vi "filter.hostToFpga.testRunner.vi"(6 "Request.Debug?":bool, 8 "error in":errorcluster, 9 "Watch.List":string[](array[string])=["AAPL"], 10 "Expected OrderBook.Command[]":T2[](array[typedef])=[{"type"=enum."AddOrder", "side"=66, "orderId "=3544385890602799695, "quantity"=20000, "symbol"=4702127773838213120, "price"=9050, "executed.qty"=0, "canceled.qty"=0, "remaining.qty"=0, "seconds"=0, "nanoseconds"=0, "Add"=FALSE, "Edit"=FALSE, "Remove"=FALSE, "seq no"=0, "recv.time"=0, "parse.time"=0}, {"type"=enum."AddOrder", "side"=66, "orderId "=3616443484640727631, "quantity"=20000, "symbol"=4702127773838213120, "price"=9050, "executed.qty"=0, "canceled.qty"=0, "remaining.qty"=0, "seconds"=0, "nanoseconds"=0, "Add"=FALSE, "Edit"=FALSE, "Remove"=FALSE, "seq no"=0, "recv.time"=0, "parse.time"=0}, {"type"=enum."AddOrder", "side"=66, "orderId "=3688501078678655567, "quantity"=20000, "symbol"=4702127773838213120, "price"=9050, "executed.qty"=0, "canceled.qty"=0, "remaining.qty"=0, "seconds"=0, "nanoseconds"=0, "Add"=FALSE, "Edit"=FALSE, "Remove"=FALSE, "seq no"=0, "recv.time"=0, "parse.time"=0}, {"type"=enum."AddOrder", "side"=66, "orderId "=3760558672716583503, "quantity"=20000, "symbol"=4702127773838213120, "price"=9050, "executed.qty"=0, "canceled.qty"=0, "remaining.qty"=0, "seconds"=0, "nanoseconds"=0, "Add"=FALSE, "Edit"=FALSE, "Remove"=FALSE, "seq no"=0, "recv.time"=0, "parse.time"=0}, {"type"=enum."AddOrder", "side"=66, "orderId "=3832616266754511439, "quantity"=20000, "symbol"=4702127773838213120, "price"=9050, "executed.qty"=0, "canceled.qty"=0, "remaining.qty"=0, "seconds"=0, "nanoseconds"=0, "Add"=FALSE, "Edit"=FALSE, "Remove"=FALSE, "seq no"=0, "recv.time"=0, "parse.time"=0}, {"type"=enum."AddOrder", "side"=66, "orderId "=3904673860792439375, "quantity"=20000, "symbol"=4702127773838213120, "price"=9050, "executed.qty"=0, "canceled.qty"=0, "remaining.qty"=0, "seconds"=0, "nanoseconds"=0, "Add"=FALSE, "Edit"=FALSE, "Remove"=FALSE, "seq no"=0, "recv.time"=0, "parse.time"=0}, {"type"=enum."AddOrder", "side"=66, "orderId "=3976731454830367311, "quantity"=20000, "symbol"=4702127773838213120, "price"=9050, "executed.qty"=0, "canceled.qty"=0, "remaining.qty"=0, "seconds"=0, "nanoseconds"=0, "Add"=FALSE, "Edit"=FALSE, "Remove"=FALSE, "seq no"=0, "recv.time"=0, "parse.time"=0}, {"type"=enum."AddOrder", "side"=66, "orderId "=4048789048868295247, "quantity"=20000, "symbol"=4702127773838213120, "price"=9050, "executed.qty"=0, "canceled.qty"=0, "remaining.qty"=0, "seconds"=0, "nanoseconds"=0, "Add"=FALSE, "Edit"=FALSE, "Remove"=FALSE, "seq no"=0, "recv.time"=0, "parse.time"=0}, {"type"=enum."AddOrder", "side"=66, "orderId "=4120846642906223183, "quantity"=20000, "symbol"=4702127773838213120, "price"=9050, "executed.qty"=0, "canceled.qty"=0, "remaining.qty"=0, "seconds"=0, "nanoseconds"=0, "Add"=FALSE, "Edit"=FALSE, "Remove"=FALSE, "seq no"=0, "recv.time"=0, "parse.time"=0}, {"type"=enum."AddOrder", "side"=66, "orderId "=4697307395209646671, "quantity"=20000, "symbol"=4702127773838213120, "price"=9050, "executed.qty"=0, "canceled.qty"=0, "remaining.qty"=0, "seconds"=0, "nanoseconds"=0, "Add"=FALSE, "Edit"=FALSE, "Remove"=FALSE, "seq no"=0, "recv.time"=0, "parse.time"=0}, {"type"=enum."AddOrder", "side"=66, "orderId "=4769364989247574607, "quantity"=20000, "symbol"=4702127773838213120, "price"=9050, "executed.qty"=0, "canceled.qty"=0, "remaining.qty"=0, "seconds"=0, "nanoseconds"=0, "Add"=FALSE, "Edit"=FALSE, "Remove"=FALSE, "seq no"=0, "recv.time"=0, "parse.time"=0}] {"symbol" format="%.0x"; "orderId" format="%.0x"; "side" format="%.0x"}, 11 "OrderBook.Commands.in":T2[](array[typedef]) {"symbol" format="%.0x"; "orderId" format="%.0x"; "side" format="%.0x"}) -> (0 "error out":errorcluster={"status"=TRUE, "code"=-61165, "source"="Open FPGA VI Reference in host.bats.parser.tester.vi"}, 1 "Data.Results.out":T4, 2 "Metadata.Results.out":T1)   [LabVIEW 2020]
uses:
  <vilib>/rvi/interface/nirviOpenFPGA/nirviOpenFPGA.xnode
  <vilib>/rvi/interface/nirviMethod/nirviMethod.xnode
  <vilib>/rvi/interface/nirviCloseFPGA/nirviCloseFPGA.xnode
  <vilib>/rvi/errors/niLvFpgaMergeErrorWithErrorCode.vi
  <vilib>/FPGAPlugInAG/Dynamic/niLvFpga_ReadFifo_Dynamic.vi
  <vilib>/rvi/interface/nirviReadWriteControl/nirviReadWriteControl.xnode
  <vilib>/rvi/interface/Simulation/niFpgaSimulationCallBeginRW.vi
  <vilib>/rvi/errors/niLvFpgaAdjustHostInterfaceError.vi
  NiFpgaLv.dll
  <vilib>/Utility/error.llb/Error Cluster From Error Code.vi
  <vilib>/FPGAPlugInAG/Dynamic/niLvFpga_WriteFifo_Dynamic.vi
  Market.Data.Common/host/fpganow.common.host.lvlib
  Market.Data.Common/fpga/orderbook.command.type.ctl
  Market.Data.Common/fpga/fpganow.common.fpga.lvlib
  Market.Data.Common/fpga/orderbook.command.ctl
  fpga/filter.test.vi
  <vilib>/FPGAPlugInAG/Dynamic/niLvFpga_Close_Dynamic.vi
  <vilib>/rvi/interface/RandomDataEmulation/nirviRandomDataOpen.vi
  <vilib>/rvi/interface/common/niFpgaCacheSessionInfoDynamic.vi
panel:
  in  "Metadata.Results":T1
  in  "Data.Results":T4
  out "Memory":u64[](array[numeric]) format="%.0x"
  out "HT-Filter.Commands.In":u64[](array[numeric])=[1, 66, 48, 20000, 4702127773838221344, 9050, 0, 0, 0, 0, 0, 0, 0, 0, 0, 0, 2, 66, 48, 0, 0, 9050, 200, 0, 0, 0, 0, 0, 0, 0, 0, 0, 5, 66, 48, 1400, 6076284164848492576, 9050, 0, 0, 0, 0, 0, 0, 0, 0, 0, 0] format="%.0x"
  out "GetState":u64[](array[numeric]) format="%.0x"
  out "Match.Details":bool[][](array[boolean])
  out "Debug.Normal.out":u64[](array[numeric]) format="%.0x"
  out "Failures.Count":i32
  out "Passed":bool
  out "OrderBook.Commands.out":T2[](array[typedef]) {"symbol" format="%.0x"; "orderId" format="%.0x"; "side" format="%.0x"}
  out "Data.size":i32
  in  "Execute?":bool=TRUE
  out "Data.out":u64[](array[numeric]) format="%.0x"
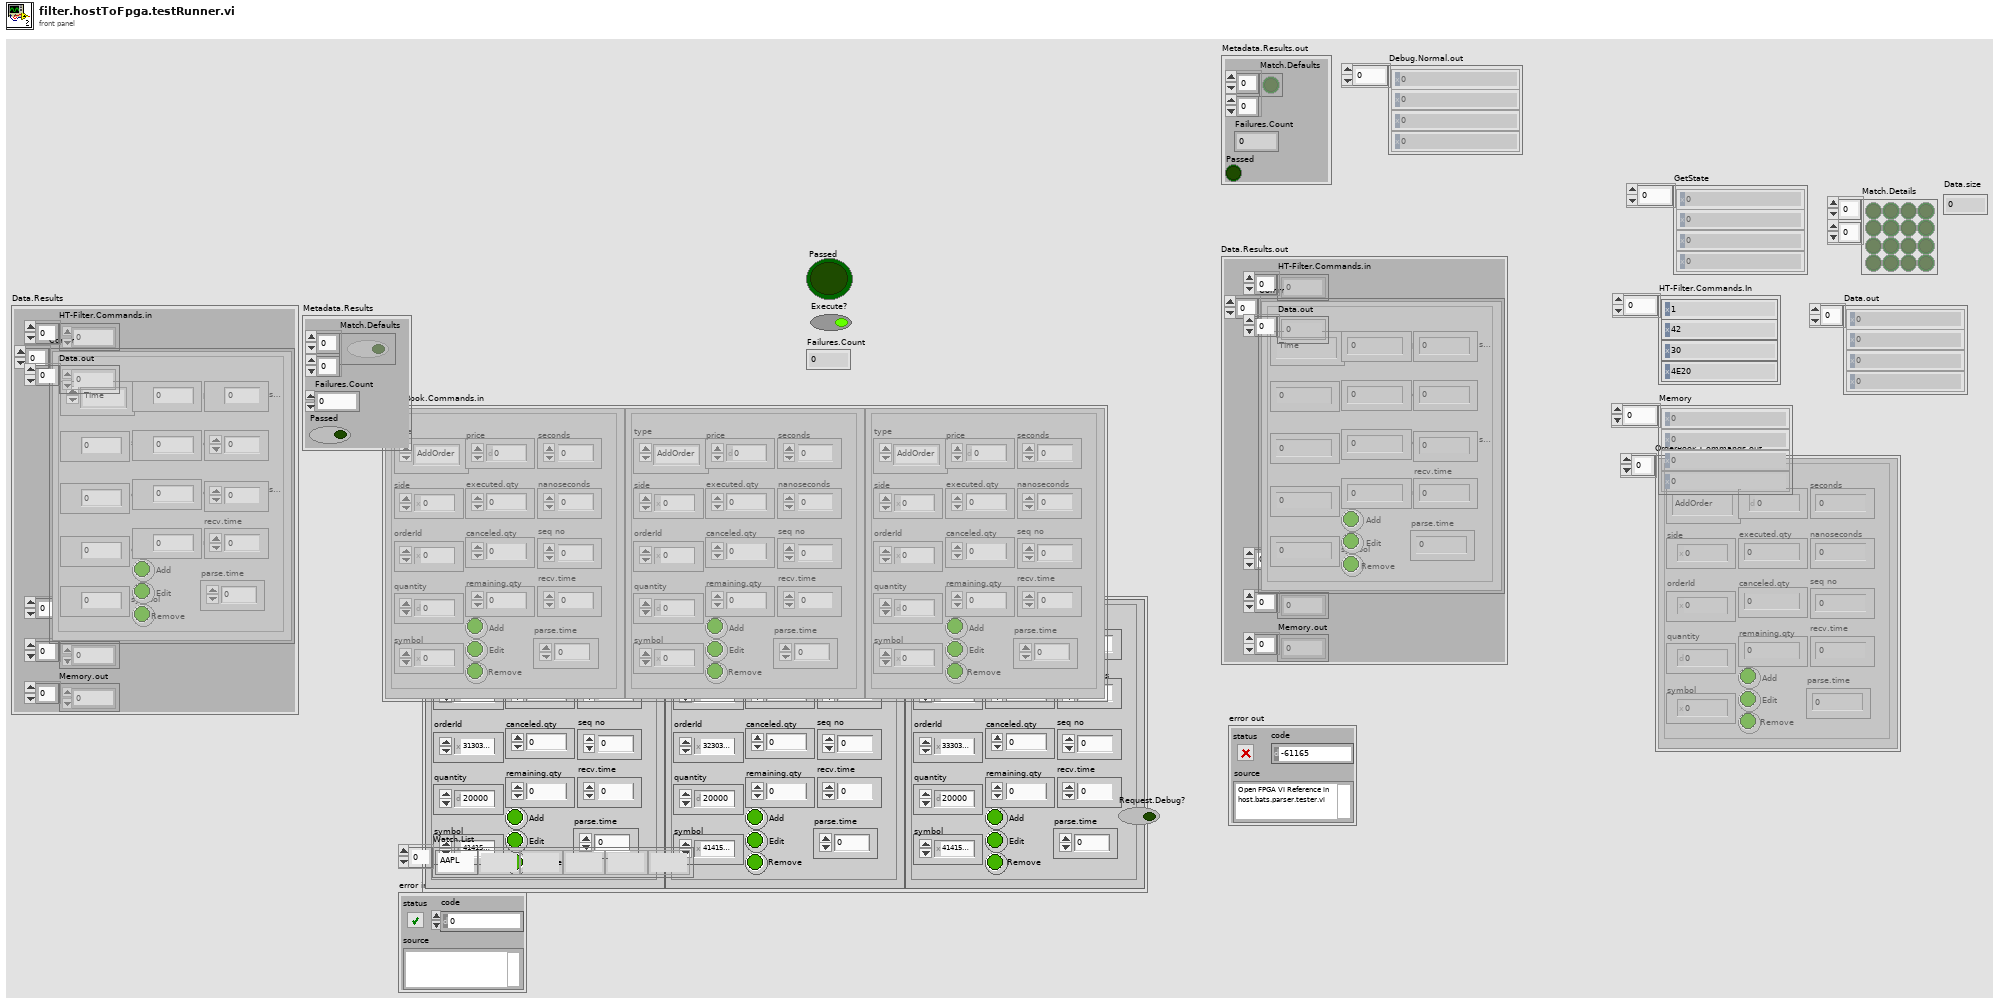
[diagram p1: front panel]
types:
  T1 = cluster{"Match.Defaults":bool[][], "Failures.Count":i32, "Passed":bool}
  T2 = typedef "fpganow.common.fpga.lvlib/orderbook.command.ctl" = cluster{"type":T3, "side":u8, "orderId ":u64, "quantity":u32, "symbol":u64, "price":u64, "executed.qty":u32, "canceled.qty":u32, "remaining.qty":u32, "seconds":u64, "nanoseconds":u64, "Add":bool, "Edit":bool, "Remove":bool, "seq no":u32, "recv.time":u64, "parse.time":u64}
  T3 = typedef "fpganow.common.fpga.lvlib/orderbook.command.type.ctl" = enum8{"Time", "AddOrder", "OrderExecuted", "OrderExecutedAtPrice", "ReduceSize", "ModifyOrder", "DeleteOrder", "Get.Everything", "Get.All.Orders", "Get.Top"}
  T4 = cluster{"HT-Filter.Commands.in":u64[], "Data.out":u64[], "Commands.out":T2[], "Debug.out":u64[], "GetState.out":u64[], "Memory.out":u64[]}
  T5 = cluster{"type":bool, "side":bool, "orderId ":bool, "quantity":bool, "symbol":bool, "price":bool, "executed.qty":bool, "canceled.qty":bool, "remaining.qty":bool, "seconds":bool, "nanoseconds":bool, "Add":bool, "Edit":bool, "Remove":bool, "Remove 2":bool}
  T6 = cluster{"Index":i32, "x = y?":cluster{"type":bool, "side":bool, "orderId ":bool, "quantity":bool, "symbol":bool, "price":bool, "executed.qty":bool, "canceled.qty":bool, "remaining.qty":bool, "seconds":bool, "nanoseconds":bool, "Add":bool, "Edit":bool, "Remove":bool, "Remove 2":bool}}
  T7 = cluster{"Index":i32, "x = y?":cluster{"type":bool, "side":bool, "orderId ":bool, "quantity":bool, "symbol":bool, "price":bool, "executed.qty":bool, "canceled.qty":bool, "remaining.qty":bool, "seconds":bool, "nanoseconds":bool, "Add":bool, "Edit":bool, "Remove":bool, "Remove 2":bool}}[]
  T8 = cluster{"type":bool, "side":bool, "orderId ":bool, "quantity":bool, "symbol":bool, "price":bool, "executed.qty":bool, "canceled.qty":bool, "remaining.qty":bool, "seconds":bool, "nanoseconds":bool, "Add":bool, "Edit":bool, "Remove":bool, "seq no":bool, "recv.time":bool, "parse.time":bool}
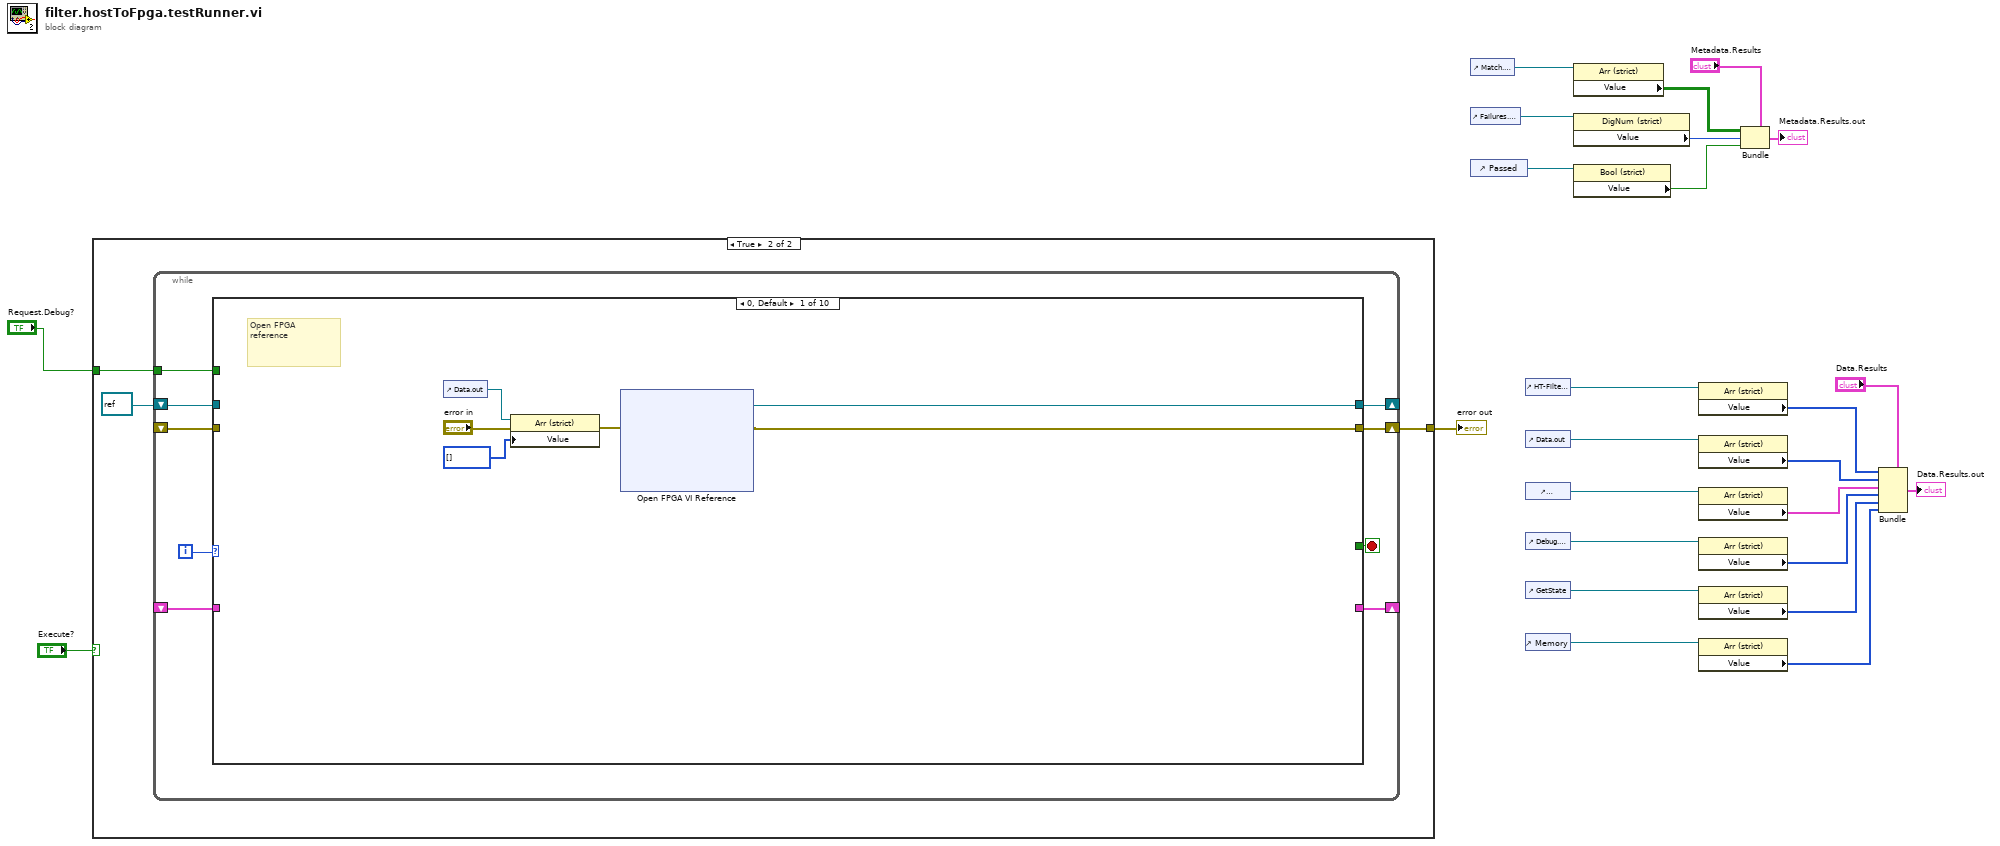
[diagram p0: block diagram]
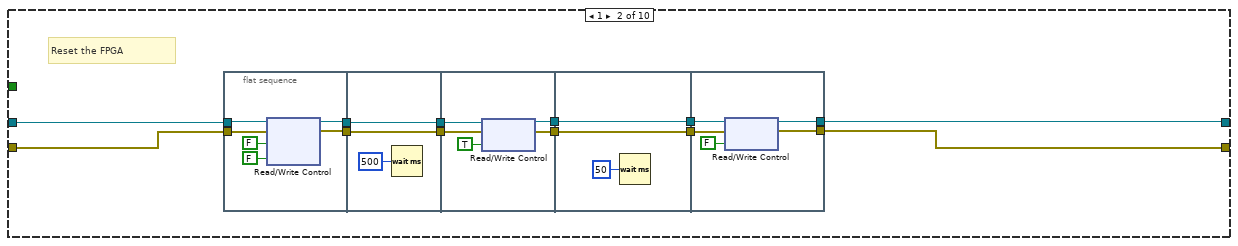
[diagram p3: hidden frame]
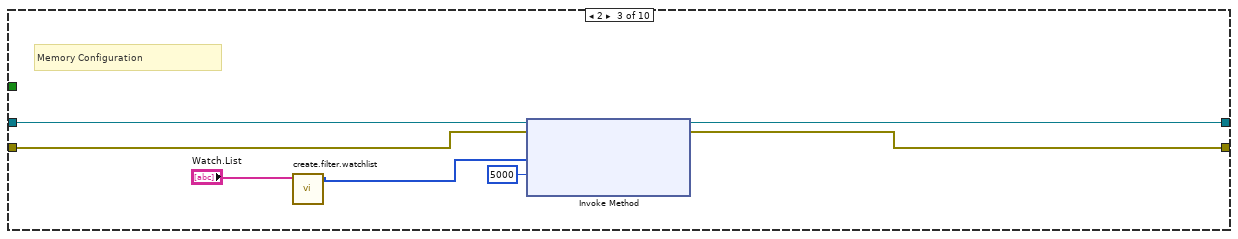
[diagram p4: hidden frame]
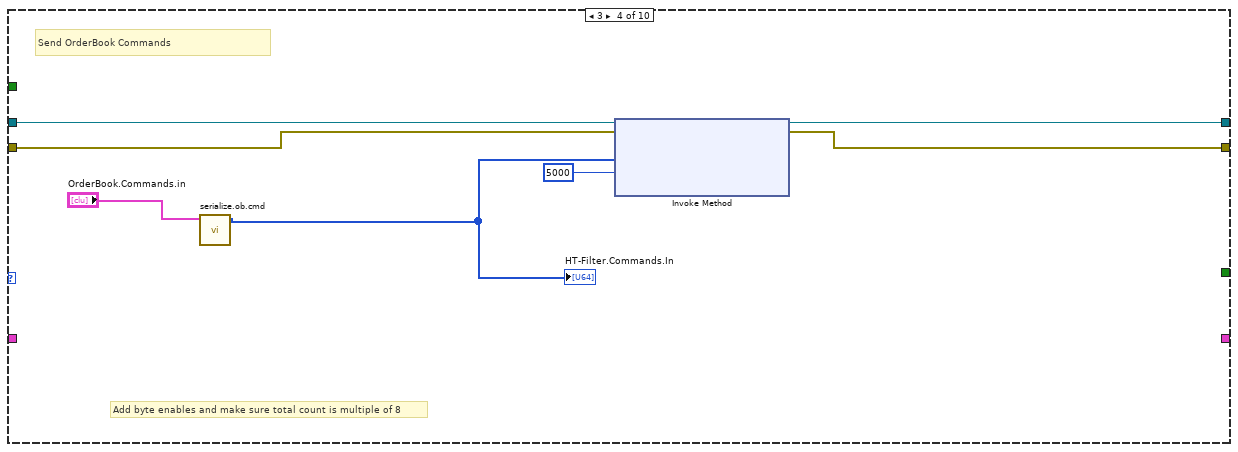
[diagram p5: hidden frame]
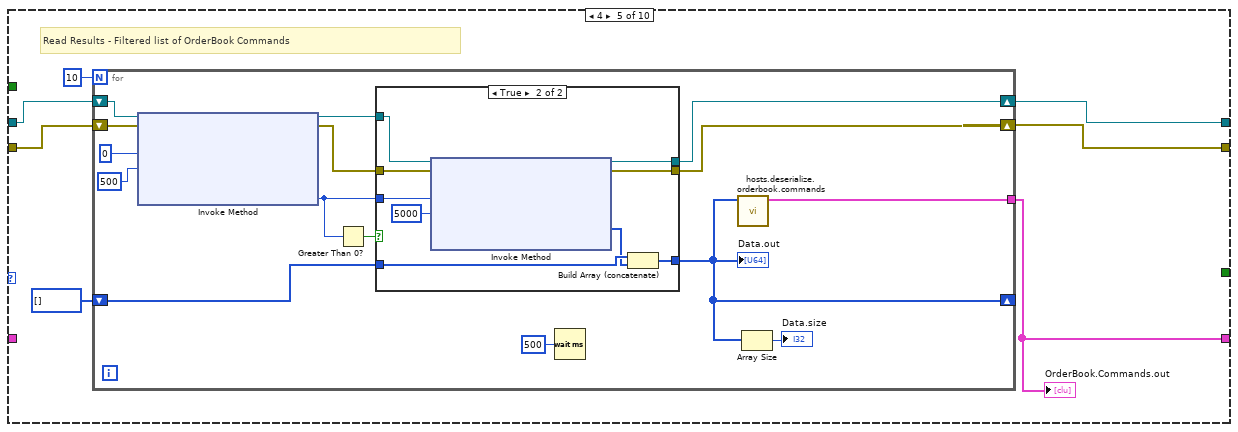
[diagram p6: hidden frame]
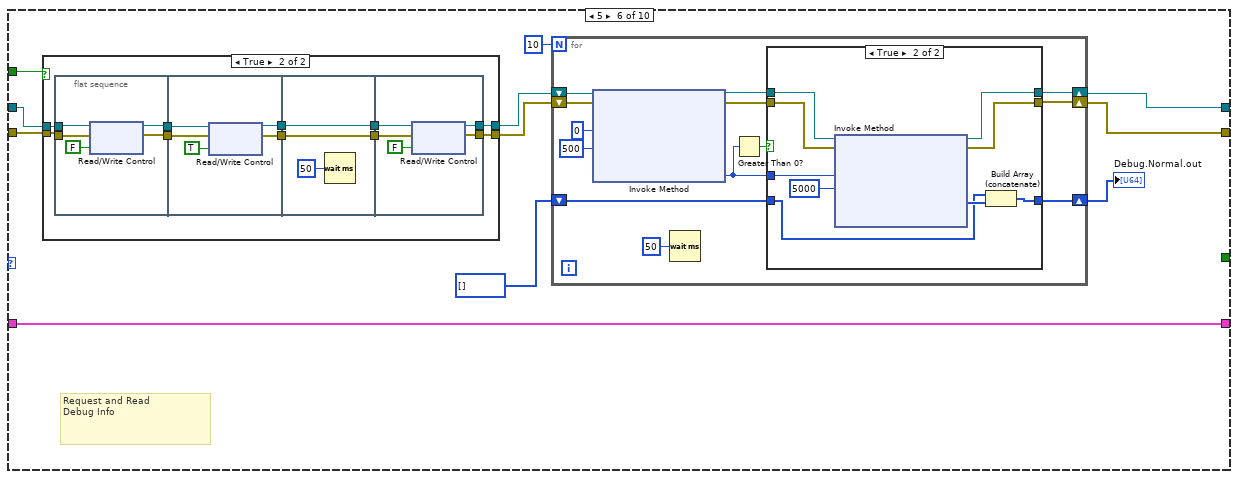
[diagram p8: hidden frame]
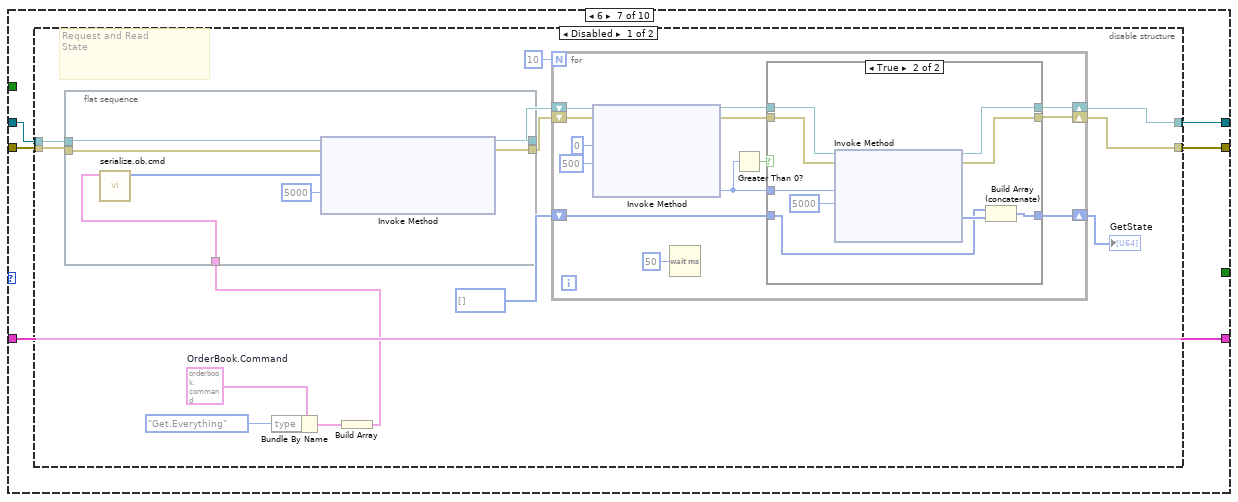
[diagram p11: hidden frame]
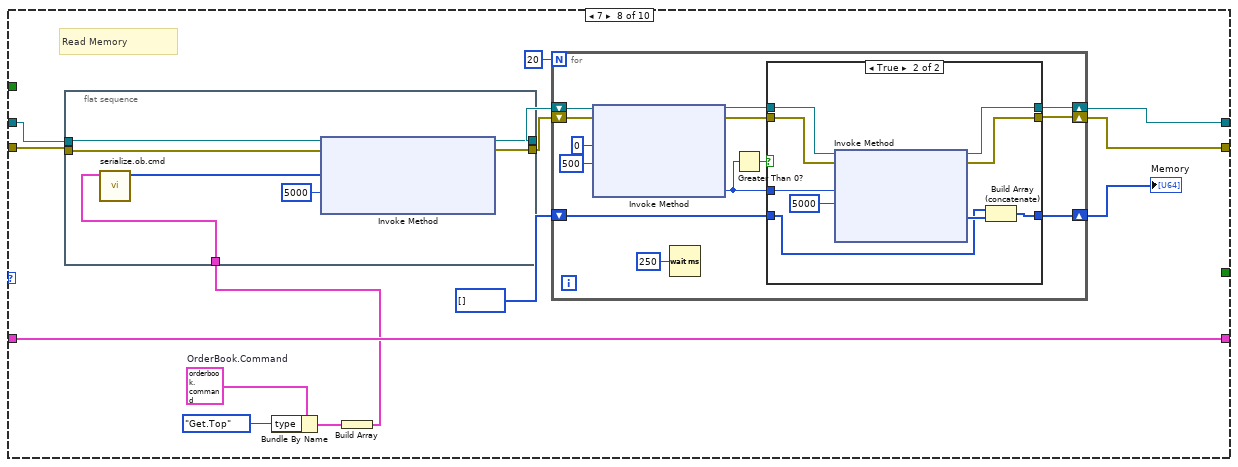
[diagram p14: hidden frame]
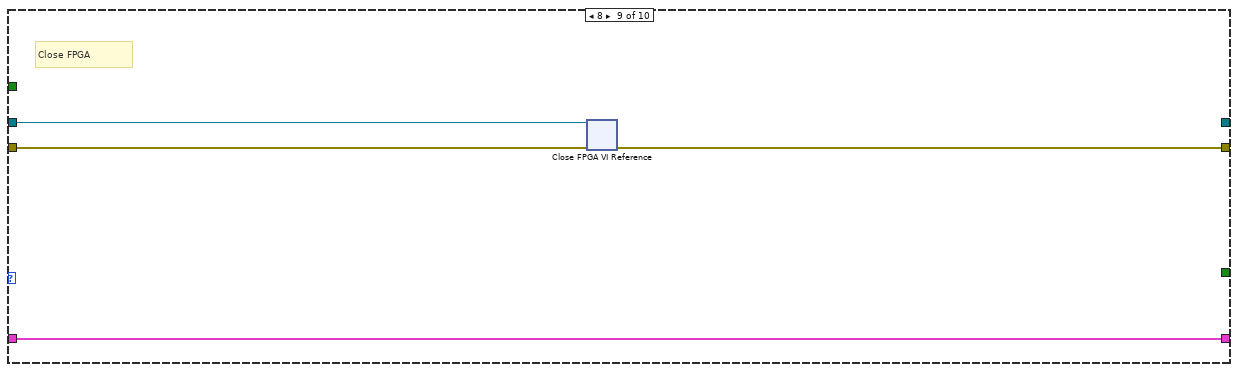
[diagram p16: hidden frame]
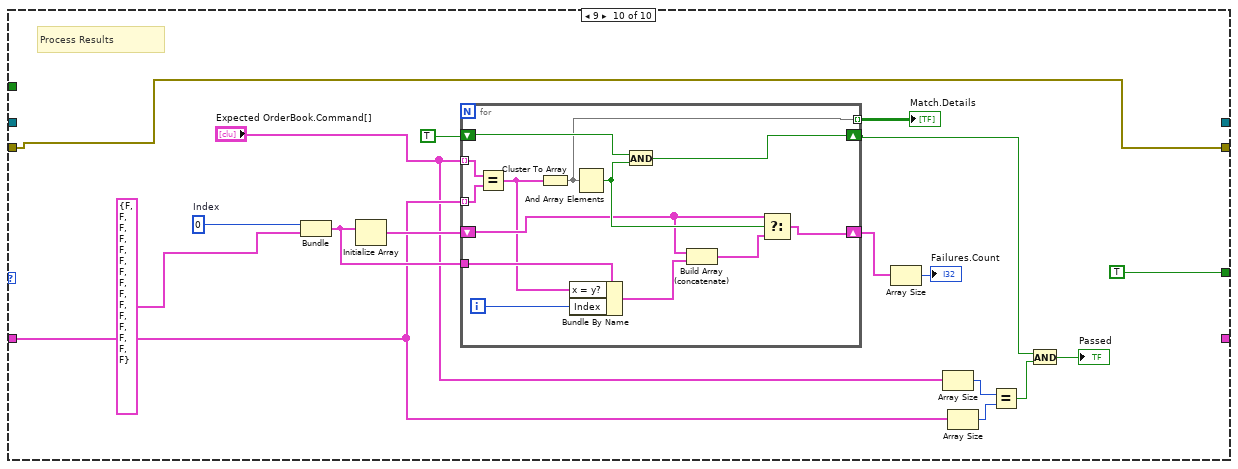
[diagram p17: hidden frame]
diagram:
  n1 = case shown="True" "Execute?" {
    tunnel: [_ w28] -> w25
    tunnel: "Request.Debug?" -> [_ w26]
    frame False {
    }
    frame True {
      n2 = while {
        shift-right: [w35] -> w28
        shift-left: _ -> [w34]
        shift-right: [w33] -> _
        shift-left: _ -> [w32]
        shift-right: [w30] -> _
        shift-left: refnum<k20> refnum ("FPGA VI Reference Out") -> [w31]
        tunnel: w26 -> [w29]
        i -> [w37]
        stop <- w36 stop-if-true
        n3 = case shown="0, Default" w37 {
          tunnel: [_ _ _ _ _ _ _ _ _ TRUE] -> w36
          tunnel: [w39 w54 w82 w90 w97 w133 w195 w256 w293 w300] -> w35
          tunnel: w34 -> [_ w55 w83 w91 w98 w136 w196 w257 w292 w300]
          tunnel: [_ _ _ _ w96 w129 w194 w255 w291 _] -> w33
          tunnel: w32 -> [_ _ _ _ _ w129 w194 w255 w291 w301]
          tunnel: [w38 w44 w78 w85 w92 w127 w192 w253 _ _] -> w30
          tunnel: w31 -> [_ w45 w79 w86 w93 w128 w193 w254 w290 _]
          tunnel: w29 -> [_ _ _ _ _ w126 _ _ _ _]
          frame 0, Default {
            # "Open FPGA\nreference"
            n4 = control-ref of="Data.out"() -> (w41:refnum<vi>)
            n5 = property class="Arr (strict)"(reference=w41, error in="error in", "Value"=u8[] []) -> (error out=w43:errorcluster)  [unwired: 1 out]
            n6 = xnode ("Open FPGA VI Reference")("error in"=w43) -> ("FPGA VI Reference Out"=w38:refnum<k20>, "error out"=w39:errorcluster)  [unwired: 1 in]
          }
          frame 1 {
            # "Reset the FPGA"
            n7 = flat-sequence {
              tunnel: w45 -> [w58]
              tunnel: w55 -> [w59]
              tunnel: [w60] -> w53
              tunnel: [w61] -> w51
              tunnel: w53 -> [w64]
              tunnel: [w64] -> w52
              tunnel: w51 -> [w63]
              tunnel: [w63] -> w50
              tunnel: [w68] -> w47
              tunnel: [w67] -> w49
              tunnel: w52 -> [w66]
              tunnel: w50 -> [w65]
              tunnel: w49 -> [w72]
              tunnel: [w72] -> w48
              tunnel: w47 -> [w71]
              tunnel: [w71] -> w46
              tunnel: [w74] -> w54
              tunnel: [w73] -> w44
              tunnel: w48 -> [w75]
              tunnel: w46 -> [w76]
              frame #0 {
                n8 = xnode "Read/Write Control"("FPGA VI Reference In"=w58, "error in"=w59, "reset"=FALSE, "debug"=FALSE) -> ("FPGA VI Reference Out"=w61:refnum<k20>, "error out"=w60:errorcluster)
              }
              frame #1 {
                n9 = Wait (ms)(milliseconds to wait=u32 500) -> ()  [unwired: 1 out]
              }
              frame #2 {
                n10 = xnode "Read/Write Control"("FPGA VI Reference In"=w65, "error in"=w66, "reset"=TRUE) -> ("FPGA VI Reference Out"=w67:refnum<k20>, "error out"=w68:errorcluster)
              }
              frame #3 {
                n11 = Wait (ms)(milliseconds to wait=u32 50) -> ()  [unwired: 1 out]
              }
              frame #4 {
                n12 = xnode "Read/Write Control"("FPGA VI Reference In"=w75, "error in"=w76, "reset"=FALSE) -> ("FPGA VI Reference Out"=w73:refnum<k20>, "error out"=w74:errorcluster)
              }
            }
          }
          frame 2 {
            # "Memory Configuration"
            n13 = call "create.filter.watchlist.vi"("watch.list"="Watch.List") -> ("memory.config"=w80:u64[])  [unwired: 10 in]
            n14 = xnode "Invoke Method"("FPGA VI Reference In"=w79, "error in"=w83, "Data"=w80, "Timeout (ms)"=5000) -> ("FPGA VI Reference Out"=w78:refnum<k20>, "error out"=w82:errorcluster)  [unwired: 1 out]
          }
          frame 3 {
            # "Add byte enables and make sure total count is multiple of 8"
            # "Send OrderBook Commands"
            n15 = call "serialize.ob.cmd.vi"("OrderBook.Commands.in"="OrderBook.Commands.in") -> ("Words.Out"=w88:u64[])  [unwired: 10 in]
            "HT-Filter.Commands.In" <- w88
            n16 = xnode "Invoke Method"("FPGA VI Reference In"=w86, "error in"=w91, "Data"=w88, "Timeout (ms)"=5000) -> ("FPGA VI Reference Out"=w85:refnum<k20>, "error out"=w90:errorcluster)  [unwired: 1 out]
          }
          frame 4 {
            # "Read Results - Filtered list of OrderBook Commands"
            n17 = for {
              N: 10 -> [_]
              shift-right: [w101] -> _
              shift-left: u64[] [] -> [w106]
              shift-right: [w105] -> w92
              shift-left: w93 -> [w113]
              shift-right: [w104] -> w97
              shift-left: w98 -> [w112]
              tunnel: [w99] -> w96
              n18 = xnode "Invoke Method"("FPGA VI Reference In"=w113, "error in"=w112, "Number of Elements"=u32 0, "Timeout (ms)"=500) -> ("FPGA VI Reference Out"=w107:refnum<k20>, "error out"=w103:errorcluster, "Elements Remaining"=w108:u32)  [unwired: 1 out]
              n19 = Greater Than 0?(x=w108) -> (x > 0?=w109:bool)
              n20 = case shown="True" w109 {
                tunnel: w108 -> [_ w125]
                tunnel: w107 -> [w115 w123]
                tunnel: [w116 w120] -> w101
                tunnel: w106 -> [w116 w122]
                tunnel: [w115 w119] -> w105
                tunnel: [w114 w118] -> w104
                tunnel: w103 -> [w114 w117]
                frame False {
                }
                frame True {
                  n21 = xnode "Invoke Method"("FPGA VI Reference In"=w123, "error in"=w117, "Number of Elements"=w125, "Timeout (ms)"=5000) -> ("FPGA VI Reference Out"=w119:refnum<k20>, "error out"=w118:errorcluster, "Data"=w121:u64[])  [unwired: 1 out]
                  n22 = Build Array (concatenate)(w122, w121) -> (w120:u64[])
                }
              }
              "Data.out" <- w101
              n23 = Wait (ms)(milliseconds to wait=u32 500) -> ()  [unwired: 1 out]
              n24 = call "hosts.deserialize.orderbook.commands.vi"("DataIn"=w101) -> ("OrderBook.Command[]"=w99:T2[])  [unwired: 10 in]
              n25 = Array Size(array=w101) -> (size(s)=→"Data.size":i32)
            }
            "OrderBook.Commands.out" <- w96
          }
          frame 5 {
            # "Request and Read\nDebug Info"
            n26 = case shown="True" w126 {
              tunnel: w136 -> [w137 w142]
              tunnel: [w138 w141] -> w135
              tunnel: [w137 w140] -> w134
              tunnel: w128 -> [w138 w139]
              frame False {
              }
              frame True {
                n27 = flat-sequence {
                  tunnel: w139 -> [w150]
                  tunnel: w142 -> [w151]
                  tunnel: [w152] -> w148
                  tunnel: [w153] -> w147
                  tunnel: [w157] -> w146
                  tunnel: [w156] -> w145
                  tunnel: w148 -> [w155]
                  tunnel: w147 -> [w154]
                  tunnel: [w161] -> w144
                  tunnel: w146 -> [w161]
                  tunnel: w145 -> [w160]
                  tunnel: [w160] -> w143
                  tunnel: w144 -> [w165]
                  tunnel: w143 -> [w164]
                  tunnel: [w163] -> w140
                  tunnel: [w162] -> w141
                  frame #0 {
                    n28 = xnode "Read/Write Control"("FPGA VI Reference In"=w150, "error in"=w151, "debug"=FALSE ("reset")) -> ("FPGA VI Reference Out"=w153:refnum<k20>, "error out"=w152:errorcluster)
                  }
                  frame #1 {
                    n29 = xnode "Read/Write Control"("FPGA VI Reference In"=w154, "error in"=w155, "debug"=TRUE ("reset")) -> ("FPGA VI Reference Out"=w156:refnum<k20>, "error out"=w157:errorcluster)
                  }
                  frame #2 {
                    n30 = Wait (ms)(milliseconds to wait=u32 50) -> ()  [unwired: 1 out]
                  }
                  frame #3 {
                    n31 = xnode "Read/Write Control"("FPGA VI Reference In"=w164, "error in"=w165, "debug"=FALSE ("reset")) -> ("FPGA VI Reference Out"=w162:refnum<k20>, "error out"=w163:errorcluster)
                  }
                }
              }
            }
            n32 = for {
              N: 10 -> [_]
              shift-right: [w173] -> w127
              shift-left: w135 -> [w179]
              shift-right: [w172] -> w133
              shift-left: w134 -> [w178]
              shift-right: [w174] -> w132
              shift-left: u64[] [] -> [w168]
              n33 = xnode "Invoke Method"("FPGA VI Reference In"=w179, "error in"=w178, "Number of Elements"=u32 0, "Timeout (ms)"=500) -> ("FPGA VI Reference Out"=w171:refnum<k20>, "error out"=w170:errorcluster, "Elements Remaining"=w169:u32)  [unwired: 1 out]
              n34 = Wait (ms)(milliseconds to wait=u32 50) -> ()  [unwired: 1 out]
              n35 = Greater Than 0?(x=w169) -> (x > 0?=w175:bool)
              n36 = case shown="True" w175 {
                tunnel: [w180 w190] -> w174
                tunnel: [w182 w189] -> w173
                tunnel: [w181 w188] -> w172
                tunnel: w171 -> [w182 w187]
                tunnel: w170 -> [w181 w186]
                tunnel: w169 -> [_ w185]
                tunnel: w168 -> [w180 w183]
                frame False {
                }
                frame True {
                  n37 = xnode "Invoke Method"("FPGA VI Reference In"=w187, "error in"=w186, "Number of Elements"=w185, "Timeout (ms)"=5000) -> ("FPGA VI Reference Out"=w189:refnum<k20>, "error out"=w188:errorcluster, "Data"=w191:u64[])  [unwired: 1 out]
                  n38 = Build Array (concatenate)(w183, w191) -> (w190:u64[])
                }
              }
            }
            "Debug.Normal.out" <- w132
          }
          frame 6 {
            n39 = disable-structure shown="Disabled" {
              disable-tunnel: w196 -> [w209 w242]
              disable-tunnel: [w206 w242] -> w195
              disable-tunnel: w193 -> [w200 w243]
              disable-tunnel: [w199 w243] -> w192
              frame Disabled {
                w203 = T2 {"type"=enum."AddOrder", "side"=66, "orderId "=48, "quantity"=20000, "symbol"=4702127773838221344, "price"=9050, "executed.qty"=0, "canceled.qty"=0, "remaining.qty"=0, "seconds"=0, "nanoseconds"=0, "Add"=FALSE, "Edit"=FALSE, "Remove"=FALSE, "seq no"=0, "recv.time"=0, "parse.time"=0}  # OrderBook.Command
                # "Request and Read\nState"
                n40 = flat-sequence {
                  tunnel: [w214] -> w207
                  tunnel: [w213] -> w208
                  tunnel: w200 -> [w215]
                  tunnel: w209 -> [w216]
                  tunnel: w201 -> [w210]
                  frame #0 {
                    n41 = call "serialize.ob.cmd.vi"("OrderBook.Commands.in"=w210) -> ("Words.Out"=w211:u64[])  [unwired: 10 in]
                    n42 = xnode "Invoke Method"("FPGA VI Reference In"=w215, "error in"=w216, "Data"=w211, "Timeout (ms)"=5000) -> ("FPGA VI Reference Out"=w213:refnum<k20>, "error out"=w214:errorcluster)  [unwired: 1 out]
                  }
                }
                n43 = Bundle By Name(cluster=w203, "type"=orderbook.command.type."Get.Everything" ("OrderBook Command.Type")) -> (w202:T2)
                n44 = Build Array(w202) -> (w201:T2[])
                n45 = for {
                  N: 10 -> [_]
                  shift-right: [w223] -> w199
                  shift-left: w208 -> [w229]
                  shift-right: [w222] -> w206
                  shift-left: w207 -> [w228]
                  shift-right: [w224] -> w197
                  shift-left: u64[] [] -> [w218]
                  n46 = xnode "Invoke Method"("FPGA VI Reference In"=w229, "error in"=w228, "Number of Elements"=u32 0, "Timeout (ms)"=500) -> ("FPGA VI Reference Out"=w221:refnum<k20>, "error out"=w220:errorcluster, "Elements Remaining"=w219:u32)  [unwired: 1 out]
                  n47 = Wait (ms)(milliseconds to wait=u32 50) -> ()  [unwired: 1 out]
                  n48 = Greater Than 0?(x=w219) -> (x > 0?=w225:bool)
                  n49 = case shown="True" w225 {
                    tunnel: [w230 w240] -> w224
                    tunnel: [w232 w239] -> w223
                    tunnel: [w231 w238] -> w222
                    tunnel: w221 -> [w232 w237]
                    tunnel: w220 -> [w231 w236]
                    tunnel: w219 -> [_ w235]
                    tunnel: w218 -> [w230 w233]
                    frame False {
                    }
                    frame True {
                      n50 = xnode "Invoke Method"("FPGA VI Reference In"=w237, "error in"=w236, "Number of Elements"=w235, "Timeout (ms)"=5000) -> ("FPGA VI Reference Out"=w239:refnum<k20>, "error out"=w238:errorcluster, "Data"=w241:u64[])  [unwired: 1 out]
                      n51 = Build Array (concatenate)(w233, w241) -> (w240:u64[])
                    }
                  }
                }
                "GetState" <- w197
              }
              frame Enabled {
              }
            }
          }
          frame 7 {
            w248 = T2 {"type"=enum."AddOrder", "side"=66, "orderId "=48, "quantity"=20000, "symbol"=4702127773838221344, "price"=9050, "executed.qty"=0, "canceled.qty"=0, "remaining.qty"=0, "seconds"=0, "nanoseconds"=0, "Add"=FALSE, "Edit"=FALSE, "Remove"=FALSE, "seq no"=0, "recv.time"=0, "parse.time"=0}  # OrderBook.Command
            # "Read Memory"
            n52 = flat-sequence {
              tunnel: [w262] -> w251
              tunnel: [w261] -> w252
              tunnel: w254 -> [w263]
              tunnel: w257 -> [w264]
              tunnel: w246 -> [w258]
              frame #0 {
                n53 = call "serialize.ob.cmd.vi"("OrderBook.Commands.in"=w258) -> ("Words.Out"=w259:u64[])  [unwired: 10 in]
                n54 = xnode "Invoke Method"("FPGA VI Reference In"=w263, "error in"=w264, "Data"=w259, "Timeout (ms)"=5000) -> ("FPGA VI Reference Out"=w261:refnum<k20>, "error out"=w262:errorcluster)  [unwired: 1 out]
              }
            }
            n55 = Bundle By Name(cluster=w248, "type"=orderbook.command.type."Get.Top") -> (w247:T2)
            n56 = Build Array(w247) -> (w246:T2[])
            n57 = for {
              N: 20 -> [_]
              shift-right: [w271] -> w253
              shift-left: w252 -> [w277]
              shift-right: [w270] -> w256
              shift-left: w251 -> [w276]
              shift-right: [w272] -> w244
              shift-left: u64[] [] -> [w266]
              n58 = xnode "Invoke Method"("FPGA VI Reference In"=w277, "error in"=w276, "Number of Elements"=u32 0, "Timeout (ms)"=500) -> ("FPGA VI Reference Out"=w269:refnum<k20>, "error out"=w268:errorcluster, "Elements Remaining"=w267:u32)  [unwired: 1 out]
              n59 = Wait (ms)(milliseconds to wait=u32 250) -> ()  [unwired: 1 out]
              n60 = Greater Than 0?(x=w267) -> (x > 0?=w273:bool)
              n61 = case shown="True" w273 {
                tunnel: [w278 w288] -> w272
                tunnel: [w280 w287] -> w271
                tunnel: [w279 w286] -> w270
                tunnel: w269 -> [w280 w285]
                tunnel: w268 -> [w279 w284]
                tunnel: w267 -> [_ w283]
                tunnel: w266 -> [w278 w281]
                frame False {
                }
                frame True {
                  n62 = xnode "Invoke Method"("FPGA VI Reference In"=w285, "error in"=w284, "Number of Elements"=w283, "Timeout (ms)"=5000) -> ("FPGA VI Reference Out"=w287:refnum<k20>, "error out"=w286:errorcluster, "Data"=w289:u64[])  [unwired: 1 out]
                  n63 = Build Array (concatenate)(w281, w289) -> (w288:u64[])
                }
              }
            }
            "Memory" <- w244
          }
          frame 8 {
            # "Close FPGA"
            n64 = xnode "Close FPGA VI Reference"("FPGA VI Reference In"=w290, "error in"=w292) -> ("error out"=w293:errorcluster)
          }
          frame 9 {
            w303 = 0  # Index
            # "Process Results"
            n65 = Bundle("Index"=w303, "x = y?"=T5 {"type"=FALSE, "side"=FALSE, "orderId "=FALSE, "quantity"=FALSE, "symbol"=FALSE, "price"=FALSE, "executed.qty"=FALSE, "canceled.qty"=FALSE, "remaining.qty"=FALSE, "seconds"=FALSE, "nanoseconds"=FALSE, "Add"=FALSE, "Edit"=FALSE, "Remove"=FALSE, "Remove 2"=FALSE}) -> (w305:T6)  [unwired: 1 in]
            n66 = Initialize Array(w305) -> (w304:T7)  [unwired: 1 in]
            n67 = for {
              tunnel: "Expected OrderBook.Command[]" -> [w323] mode=indexing
              tunnel: w301 -> [w322] mode=indexing
              shift-right: [w320] -> w309
              shift-left: TRUE -> [w321]
              shift-right: [w318] -> w306
              shift-left: w304 -> [w314]
              tunnel: w305 -> [w317]
              tunnel: [w312] -> w295 mode=indexing
              i -> [w316]
              n68 = Equal?(x=w323, y=w322) -> (x = y?=w311:T8)
              n69 = Cluster To Array(cluster=w311) -> (array=w312:bool[])
              n70 = Bundle By Name(cluster=w317, "x = y?"=w311, "Index"=w316) -> (w315:T6)
              n71 = And Array Elements(Boolean array=w312) -> (logical AND=w319:bool)
              n72 = And(x=w321, y=w319) -> (x .and. y?=w320:bool)
              n73 = Build Array (concatenate)(w314, w315) -> (w313:T7)
              n74 = Select(t=w314, s=w319, f=w313) -> (s? t:f=w318:T7)
            }
            "Match.Details" <- w295
            n75 = Array Size(array=w306) -> (size(s)=→"Failures.Count":i32)
            n76 = Array Size(array="Expected OrderBook.Command[]") -> (size(s)=w298:i32)
            n77 = Array Size(array=w301) -> (size(s)=w297:i32)
            n78 = Equal?(x=w298, y=w297) -> (x = y?=w296:bool)
            n79 = And(x=w309, y=w296) -> (x .and. y?=→"Passed":bool)
          }
        }
      }
    }
  }
  "error out" <- w25
  n80 = control-ref of="Match.Details"() -> (w8:refnum<vi>)
  n81 = control-ref of="Failures.Count"() -> (w7:refnum<vi>)
  n82 = control-ref of="Passed"() -> (w6:refnum<vi>)
  n83 = control-ref of="HT-Filter.Commands.In"() -> (w20:refnum<vi>)
  n84 = control-ref of="Data.out"() -> (w19:refnum<vi>)
  n85 = control-ref of="OrderBook.Commands.out"() -> (w18:refnum<vi>)
  n86 = control-ref of="Debug.Normal.out"() -> (w17:refnum<vi>)
  n87 = control-ref of="GetState"() -> (w21:refnum<vi>)
  n88 = control-ref of="Memory"() -> (w22:refnum<vi>)
  n89 = property class="Arr (strict)"(reference=w8) -> ("Value"=w5:bool[][])  [unwired: 1 in, 2 out]
  n90 = property class="DigNum (strict)"(reference=w7) -> ("Value"=w4:i32)  [unwired: 1 in, 2 out]
  n91 = property class="Bool (strict)"(reference=w6) -> ("Value"=w3:bool)  [unwired: 1 in, 2 out]
  n92 = property class="Arr (strict)"(reference=w20) -> ("Value"=w16:u64[])  [unwired: 1 in, 2 out]
  n93 = property class="Arr (strict)"(reference=w19) -> ("Value"=w15:u64[])  [unwired: 1 in, 2 out]
  n94 = property class="Arr (strict)"(reference=w18) -> ("Value"=w14:T2[])  [unwired: 1 in, 2 out]
  n95 = property class="Arr (strict)"(reference=w17) -> ("Value"=w13:u64[])  [unwired: 1 in, 2 out]
  n96 = property class="Arr (strict)"(reference=w21) -> ("Value"=w12:u64[])  [unwired: 1 in, 2 out]
  n97 = property class="Arr (strict)"(reference=w22) -> ("Value"=w11:u64[])  [unwired: 1 in, 2 out]
  n98 = Bundle(cluster="Metadata.Results", "Match.Defaults"=w5, "Failures.Count"=w4, "Passed"=w3) -> (→"Metadata.Results.out":T1)
  n99 = Bundle(cluster="Data.Results", "HT-Filter.Commands.in"=w16, "Data.out"=w15, "Commands.out"=w14, "Debug.out"=w13, "GetState.out"=w12, "Memory.out"=w11) -> (→"Data.Results.out":T4)
